vi "movimentacao_cin_inv_bezier_2.vi"() -> ()   [LabVIEW 2017]
doc: "The myRIO Project template acquires acceleration data from the onboard accelerometer and displays the changes of acceleration values in a waveform chart."
uses:
  <vilib>/Analysis/Matrix/Datatypes/RealMatrix.ctl
  <vilib>/myRIO/Instrument Drivers/Onboard IO/I2C/typedefs/I2C User Configuration.ctl
  <vilib>/myRIO/Instrument Drivers/Onboard IO/I2C/typedefs/I2C Transfer Rate.ctl
  <vilib>/myRIO/Instrument Drivers/Onboard IO/PWM/typedefs/PWM Reference.ctl
  <vilib>/myRIO/Common/Instrument Driver Framework/Utilities/typedefs/myRIO Generic Hardware Reference.ctl
  <vilib>/myRIO/Common/Instrument Driver Framework/Utilities/typedefs/Hardware Version Enum.ctl
  <vilib>/myRIO/Common/Instrument Driver Framework/Utilities/typedefs/myRIO v1.0 Reference.ctl
  <vilib>/myRIO/Common/Instrument Driver Framework/Utilities/typedefs/Generic FPGA Reference.ctl
  <vilib>/myRIO/Common/Instrument Driver Framework/myRIO v1.0/PWM/typedefs/PWM Channels Enum.ctl
  <vilib>/myRIO/Instrument Drivers/Onboard IO/PWM/typedefs/PWM Configuration.ctl
  <vilib>/userdefined/High Color/nirio_resource_hc.ctl
  <vilib>/myRIO/Instrument Drivers/Onboard IO/I2C/typedefs/I2C Reference.ctl
  <vilib>/myRIO/Common/Instrument Driver Framework/myRIO v1.0/I2C/typedefs/I2C Channels Enum.ctl
  <vilib>/myRIO/Instrument Drivers/Onboard IO/I2C/typedefs/I2C Configuration.ctl
  <vilib>/myRIO/Common/Instrument Driver Framework/myRIO v1.0/I2C/vis/myRIO v1.1 Open I2C.vi
  <vilib>/myRIO/Common/Instrument Driver Framework/myRIO v1.0/PWM/vis/myRIO v1.1 Open PWM.vi
  <vilib>/myRIO/Common/Instrument Driver Framework/Utilities/vis/Validate Channels.vi
  <vilib>/myRIO/Common/Instrument Driver Framework/myRIO v1.0/I2C/vis/myRIO v1.0 Reserve I2C.vi
  <vilib>/myRIO/Common/Instrument Driver Framework/myRIO v1.0/PWM/vis/myRIO v1.0 Reserve PWM.vi
  <vilib>/myRIO/Instrument Drivers/Onboard IO/PWM/vis/Set Duty Cycle and Frequency.vi
  <vilib>/myRIO/Common/Instrument Driver Framework/myRIO v1.0/I2C/vis/myRIO v1.0 Close I2C.vi
  <vilib>/myRIO/Common/Instrument Driver Framework/myRIO v1.0/PWM/vis/myRIO v1.0 Close PWM.vi
  <vilib>/myRIO/Common/Instrument Driver Framework/myRIO v1.0/I2C/vis/myRIO v1.0 Build MUX Configuration I2C.vi
  <vilib>/myRIO/Common/Instrument Driver Framework/myRIO v1.0/Resource Manager/vis/myRIO v1.0 Reserve Channel List.vi
  <vilib>/myRIO/Common/Instrument Driver Framework/myRIO v1.0/PWM/vis/myRIO v1.0 Build MUX Configuration PWM.vi
  <vilib>/myRIO/Common/Instrument Driver Framework/myRIO v1.0/I2C/vis/myRIO v1.0 Unreserve I2C.vi
  <vilib>/myRIO/Common/Instrument Driver Framework/myRIO v1.0/PWM/vis/myRIO v1.0 Unreserve PWM.vi
  <vilib>/myRIO/Common/Instrument Driver Framework/myRIO v1.0/Resource Manager/vis/myRIO v1.0 Create Configuration List.vi
  <vilib>/myRIO/Common/Instrument Driver Framework/myRIO v1.0/Resource Manager/vis/myRIO v1.0 Reserve Channel.vi
  <vilib>/myRIO/Common/Instrument Driver Framework/myRIO v1.0/Resource Manager/vis/myRIO v1.0 Unreserve Channel.vi
  <vilib>/myRIO/Common/Instrument Driver Framework/myRIO v1.0/Resource Manager/vis/myRIO v1.0 Unreserve Channel List.vi
  <vilib>/myRIO/Common/Instrument Driver Framework/myRIO v1.0/Resource Manager/vis/myRIO v1.0 Build Mutex Name.vi
  <vilib>/Utility/VariantDataType/GetNumericInfo.vi
  <vilib>/Utility/error.llb/Error Cluster From Error Code.vi
  <vilib>/myRIO/Common/Instrument Driver Framework/myRIO v1.0/myRIO v1.1 Open.vi
  <vilib>/myRIO/Common/Instrument Driver Framework/Utilities/vis/IO Manager.vi
  <vilib>/myRIO/Common/Instrument Driver Framework/Utilities/vis/Configuration Manager.vi
  <vilib>/myRIO/Common/Instrument Driver Framework/myRIO v1.0/Resource Manager/vis/myRIO v1.0 Configure IO.vi
  <vilib>/myRIO/Common/Instrument Driver Framework/myRIO v1.0/myRIO v1.0 Close.vi
  <vilib>/myRIO/Common/Instrument Driver Framework/myRIO v1.0/PWM/vis/myRIO v1.0 Write PWM.vi
  <vilib>/myRIO/Common/Instrument Driver Framework/myRIO v1.0/I2C/vis/myRIO v1.0 Configure I2C.vi
  <vilib>/myRIO/Common/Instrument Driver Framework/myRIO v1.0/I2C/vis/myRIO v1.0 Shutdown I2C.vi
  <vilib>/myRIO/Common/Instrument Driver Framework/myRIO v1.0/PWM/vis/myRIO v1.0 Shutdown PWM.vi
  <vilib>/myRIO/Instrument Drivers/Onboard IO/PWM/vis/myRIO PWM Open.xnode
  <vilib>/myRIO/Instrument Drivers/Onboard IO/I2C/vis/myRIO I2C Open.xnode
  <vilib>/myRIO/Instrument Drivers/Onboard IO/PWM/PWM.lvlib
  <vilib>/myRIO/Instrument Drivers/Onboard IO/I2C/I2C.lvlib
  <vilib>/Analysis/Matrix/NI_Matrix.lvlib
panel:
  out "Range":u16
  out "Waveform Chart":u16(graph)
  out "Objeto":bool
  out "did_timeout":bool
  out "dt":u32
  out "distancaia":dbl format="%0.2f"
  out "error out":errorcluster
  out "init status":bool
  out "Objeto detectado 2":bool
  out "Parar_esteira":bool
  out "result string":string
  out "iterador":u32
  out "number of rows":i32
  out "matrix":T1
  in  "Ring":u16(ring) items=["A", "B", "C"]
  out "x .and. y?":bool
  in  "OK Button":bool
  out "subarray":dbl[](array[numeric])
  out "appended array 2":dbl[](array[numeric])
  out "logical AND":bool
  out "x = y?":bool[](array[boolean])
  out "POS_E_ORIEN_HOME":dbl[](array[numeric])
  out "ANG_POSI_E_ORIEN_HOME":dbl[](array[numeric])
  out "CURRENT POSITIONS OF THE MOTORS":dbl[](array[numeric])
  in  "angulo_garra":dbl(knob) scale=-180.0..180.0
  in  "Duty Cycle Abert":dbl=0.04 format="%#_13g"
  out "Actuator 2":bool
  in  "Actuator":bool
  in  "Conveyor speed (mm/s)":dbl(slide)=200.0 step=1.0 scale=0.0..350.0
  out "indexador":i32
  out "Objeto detectado":bool
  out "Manipulando":bool
  out "Está em Home":bool
  out "Posicao_desejada":bool
  in  "Home":bool
  in  "error in (no error)":errorcluster
  in  "PARAR":bool
  in  "POSITION VECTOR":dbl[](array[numeric])
  # "ROTINA DE CONTROLE DO PROTÓTIPO DE FMS"
  # "COMANDO DE POSIÇÃO\nATUAL DOS MOTORES"
  # "OPERATION STATUS"
  # "ÂNGULOS DE JUNTAS"
  # "THETA 1"
  # "MOTOR 1"
  # "HOME"
  # "THETA 2"
  # "MOTOR 2"
  # "DESIRED POSITION"
  # "THETA 3"
  # "MOTOR 3"
  # "OBJECT DETECTED"
  # "THETA 4"
  # "MOTOR 4"
  # "MANIPULATING"
  # "THETA 5"
  # "MOTOR 5"
  # "ACTUATOR"
  # "MOTOR 6"
  # "VELOCIDADE DA ESTEIRA (mm/s)"
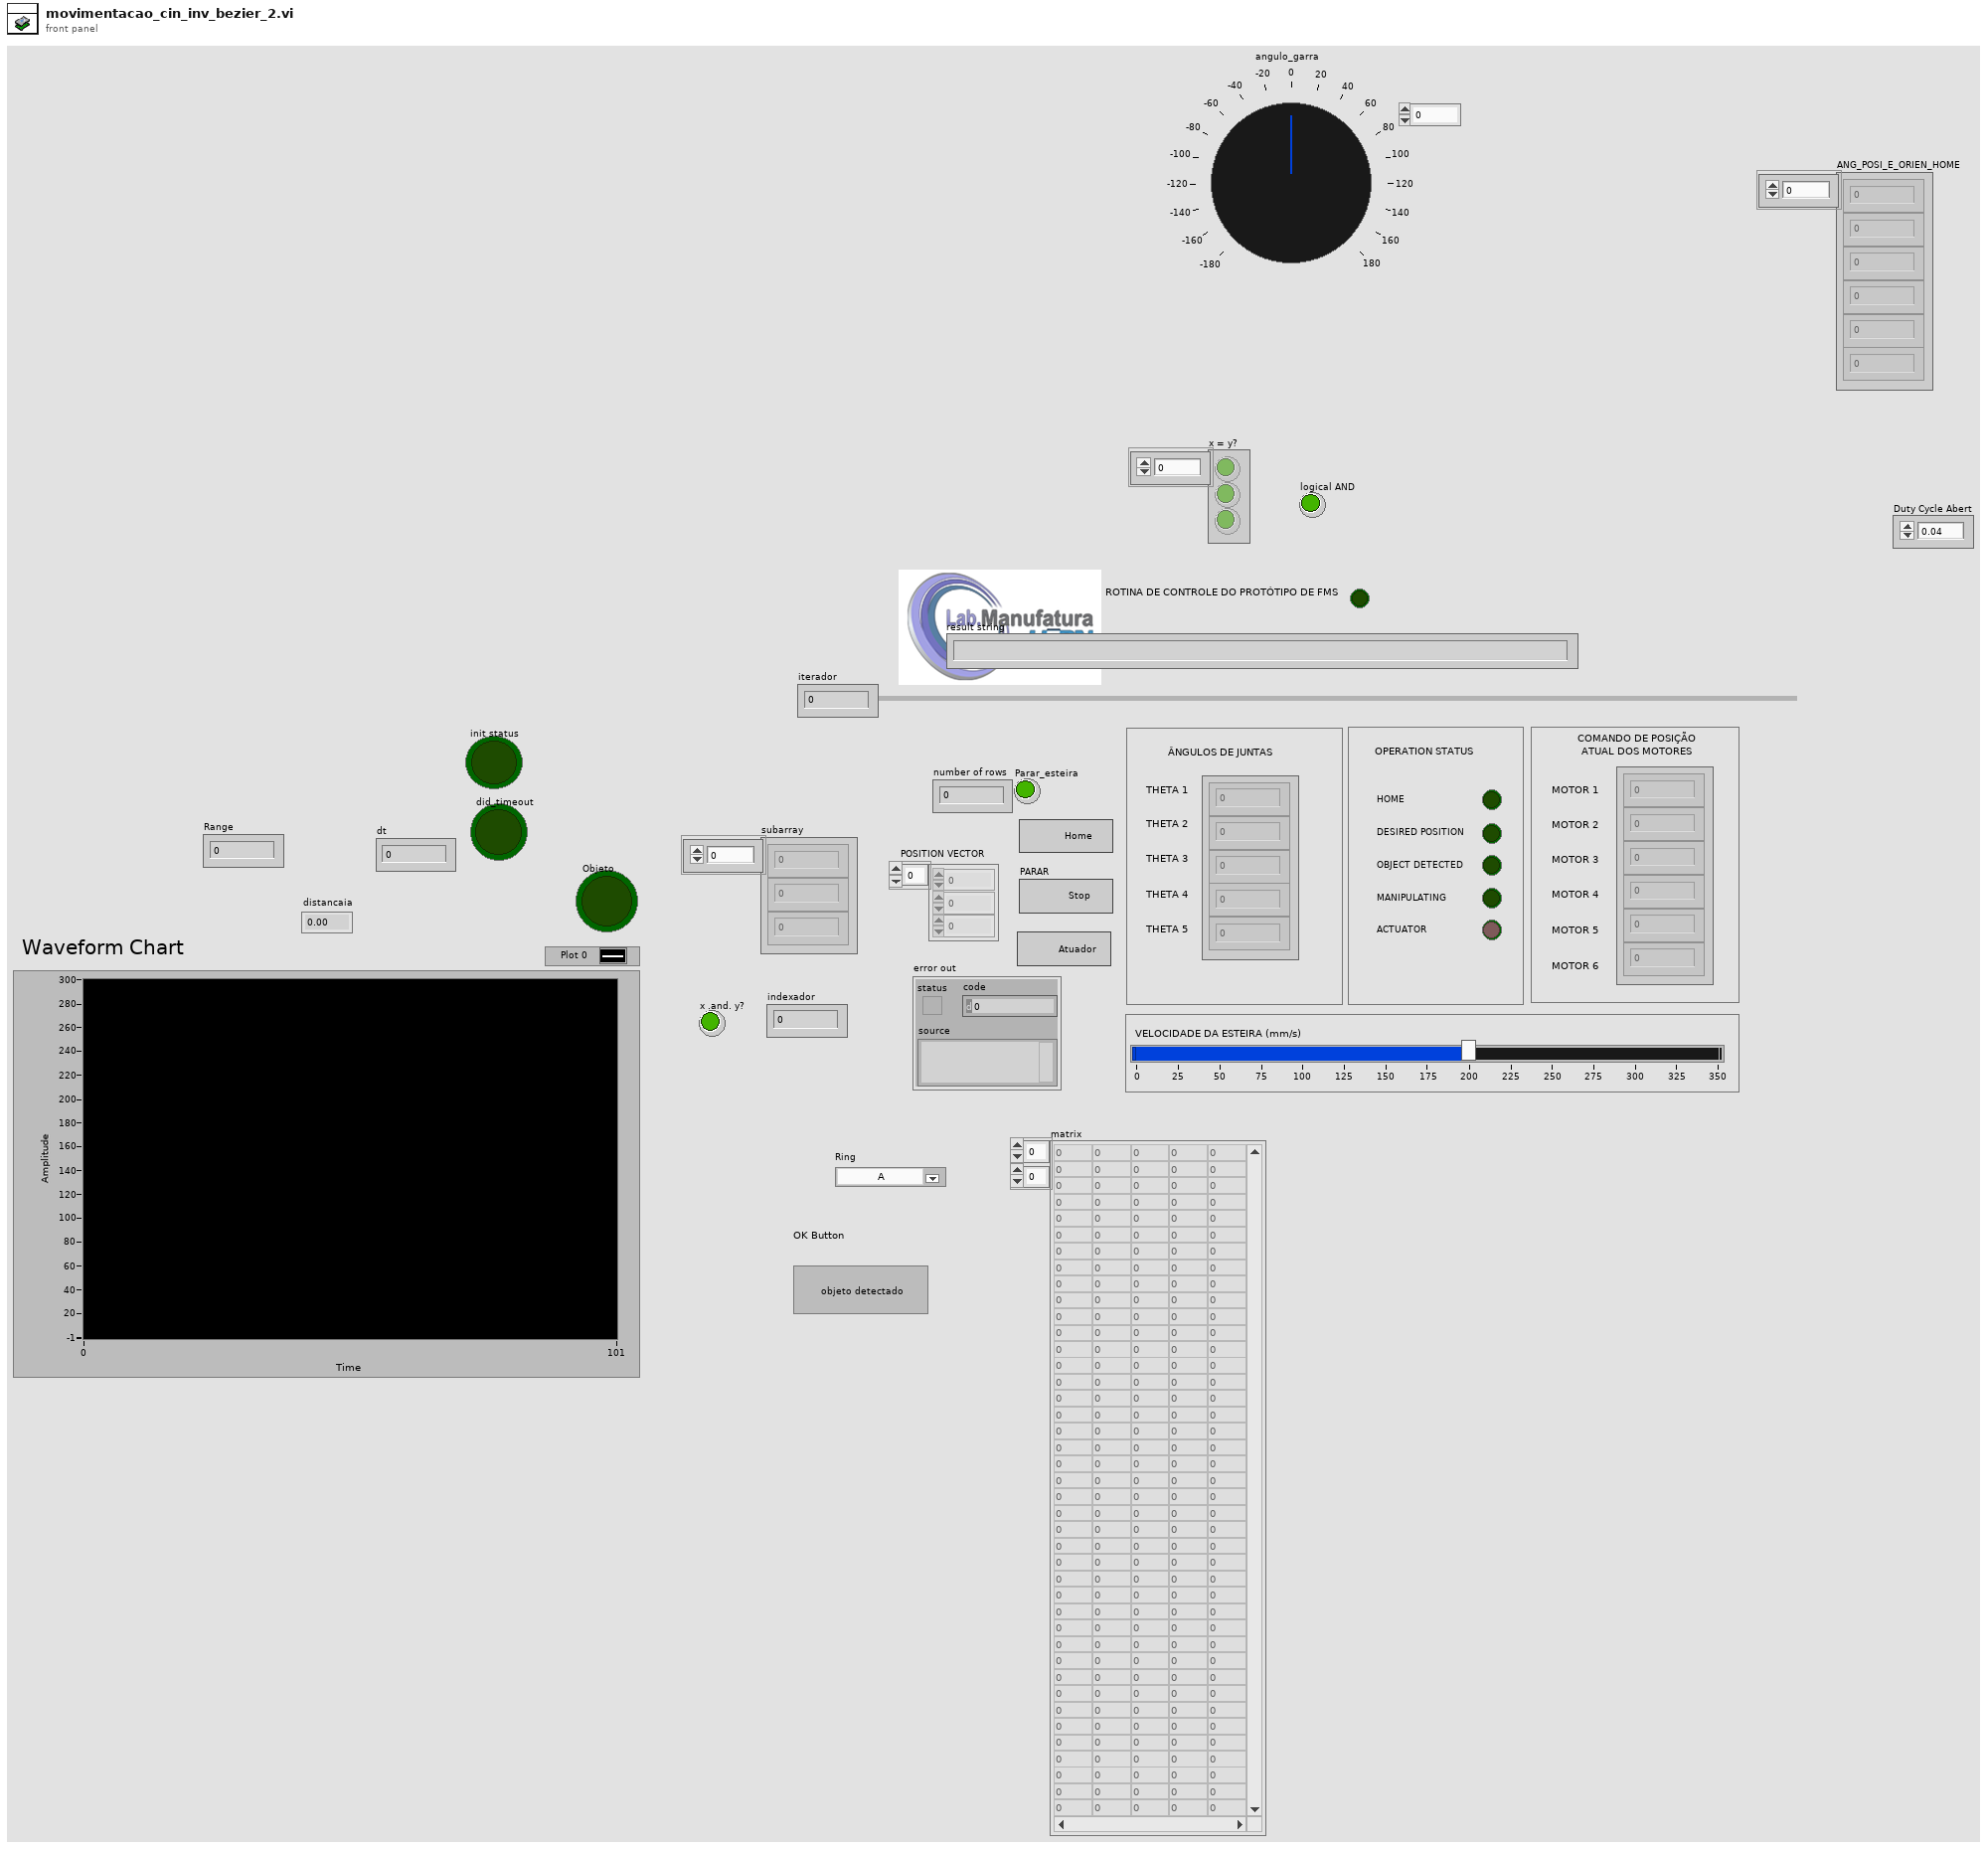
[diagram p1: front panel]
types:
  T1 = typedef "NI_Matrix.lvlib/RealMatrix.ctl" = dbl[][]
  T2 = typedef "I2C.lvlib/I2C User Configuration.ctl" = cluster{"I2C Transfer Rate":T3}
  T3 = typedef "I2C.lvlib/I2C Transfer Rate.ctl" = enum16{"Standard mode (100 kbps)", "Fast mode (400 kbps)"}
  T4 = cluster{"theta 1":dbl, "theta 2":dbl, "theta 3":dbl, "theta5":dbl, "theta4":dbl}
  T5 = typedef "I2C.lvlib/I2C Reference.ctl" = cluster{"myRIO Reference":T6, "I2C Channels Enum":T10, "I2C Configuration":T11}
  T6 = typedef "myRIO Generic Hardware Reference.ctl" = cluster{"myRIO Model":T7, "myRIO Hardware Reference":T8}
  T7 = typedef "Hardware Version Enum.ctl" = enum16{"Unknown", "myRIO-1900", "myRIO-1950", "roboRIO", "NI ELVIS RIO CM"}
  T8 = typedef "myRIO v1.0 Reference.ctl" = cluster{"Generic FPGA Reference":T9, "Allow multiple opens":bool}
  T9 = typedef "Generic FPGA Reference.ctl" = refnum<k20>
  T10 = typedef "I2C Channels Enum.ctl" = enum16{"Not Connected", "A/I2C", "B/I2C", "I2C/I2C"}
  T11 = typedef "I2C.lvlib/I2C Configuration.ctl" = cluster{"I2C Transfer Rate":T3}
  T12 = typedef "nirio_resource_hc.ctl" = tag
  T13 = typedef "PWM.lvlib/PWM Reference.ctl" = cluster{"myRIO Reference":T6, "PWM Channels Enum":T14, "PWM Configuration":T15}
  T14 = typedef "PWM Channels Enum.ctl" = enum16{"Not Connected", "C/PWM0", "C/PWM1", "A/PWM0", "A/PWM1", "A/PWM2", "B/PWM0", "B/PWM1", "B/PWM2", "PWM/PWM0", "PWM/PWM1", "PWM/PWM2", "PWM/PWM3", "PWM/PWM4", "PWM/PWM5", "PWM/PWM6", "PWM/PWM7", "PWM/PWM8", "PWM/PWM9"}
  T15 = typedef "PWM.lvlib/PWM Configuration.ctl" = cluster{"Frequency":dbl, "Duty Cycle":dbl}
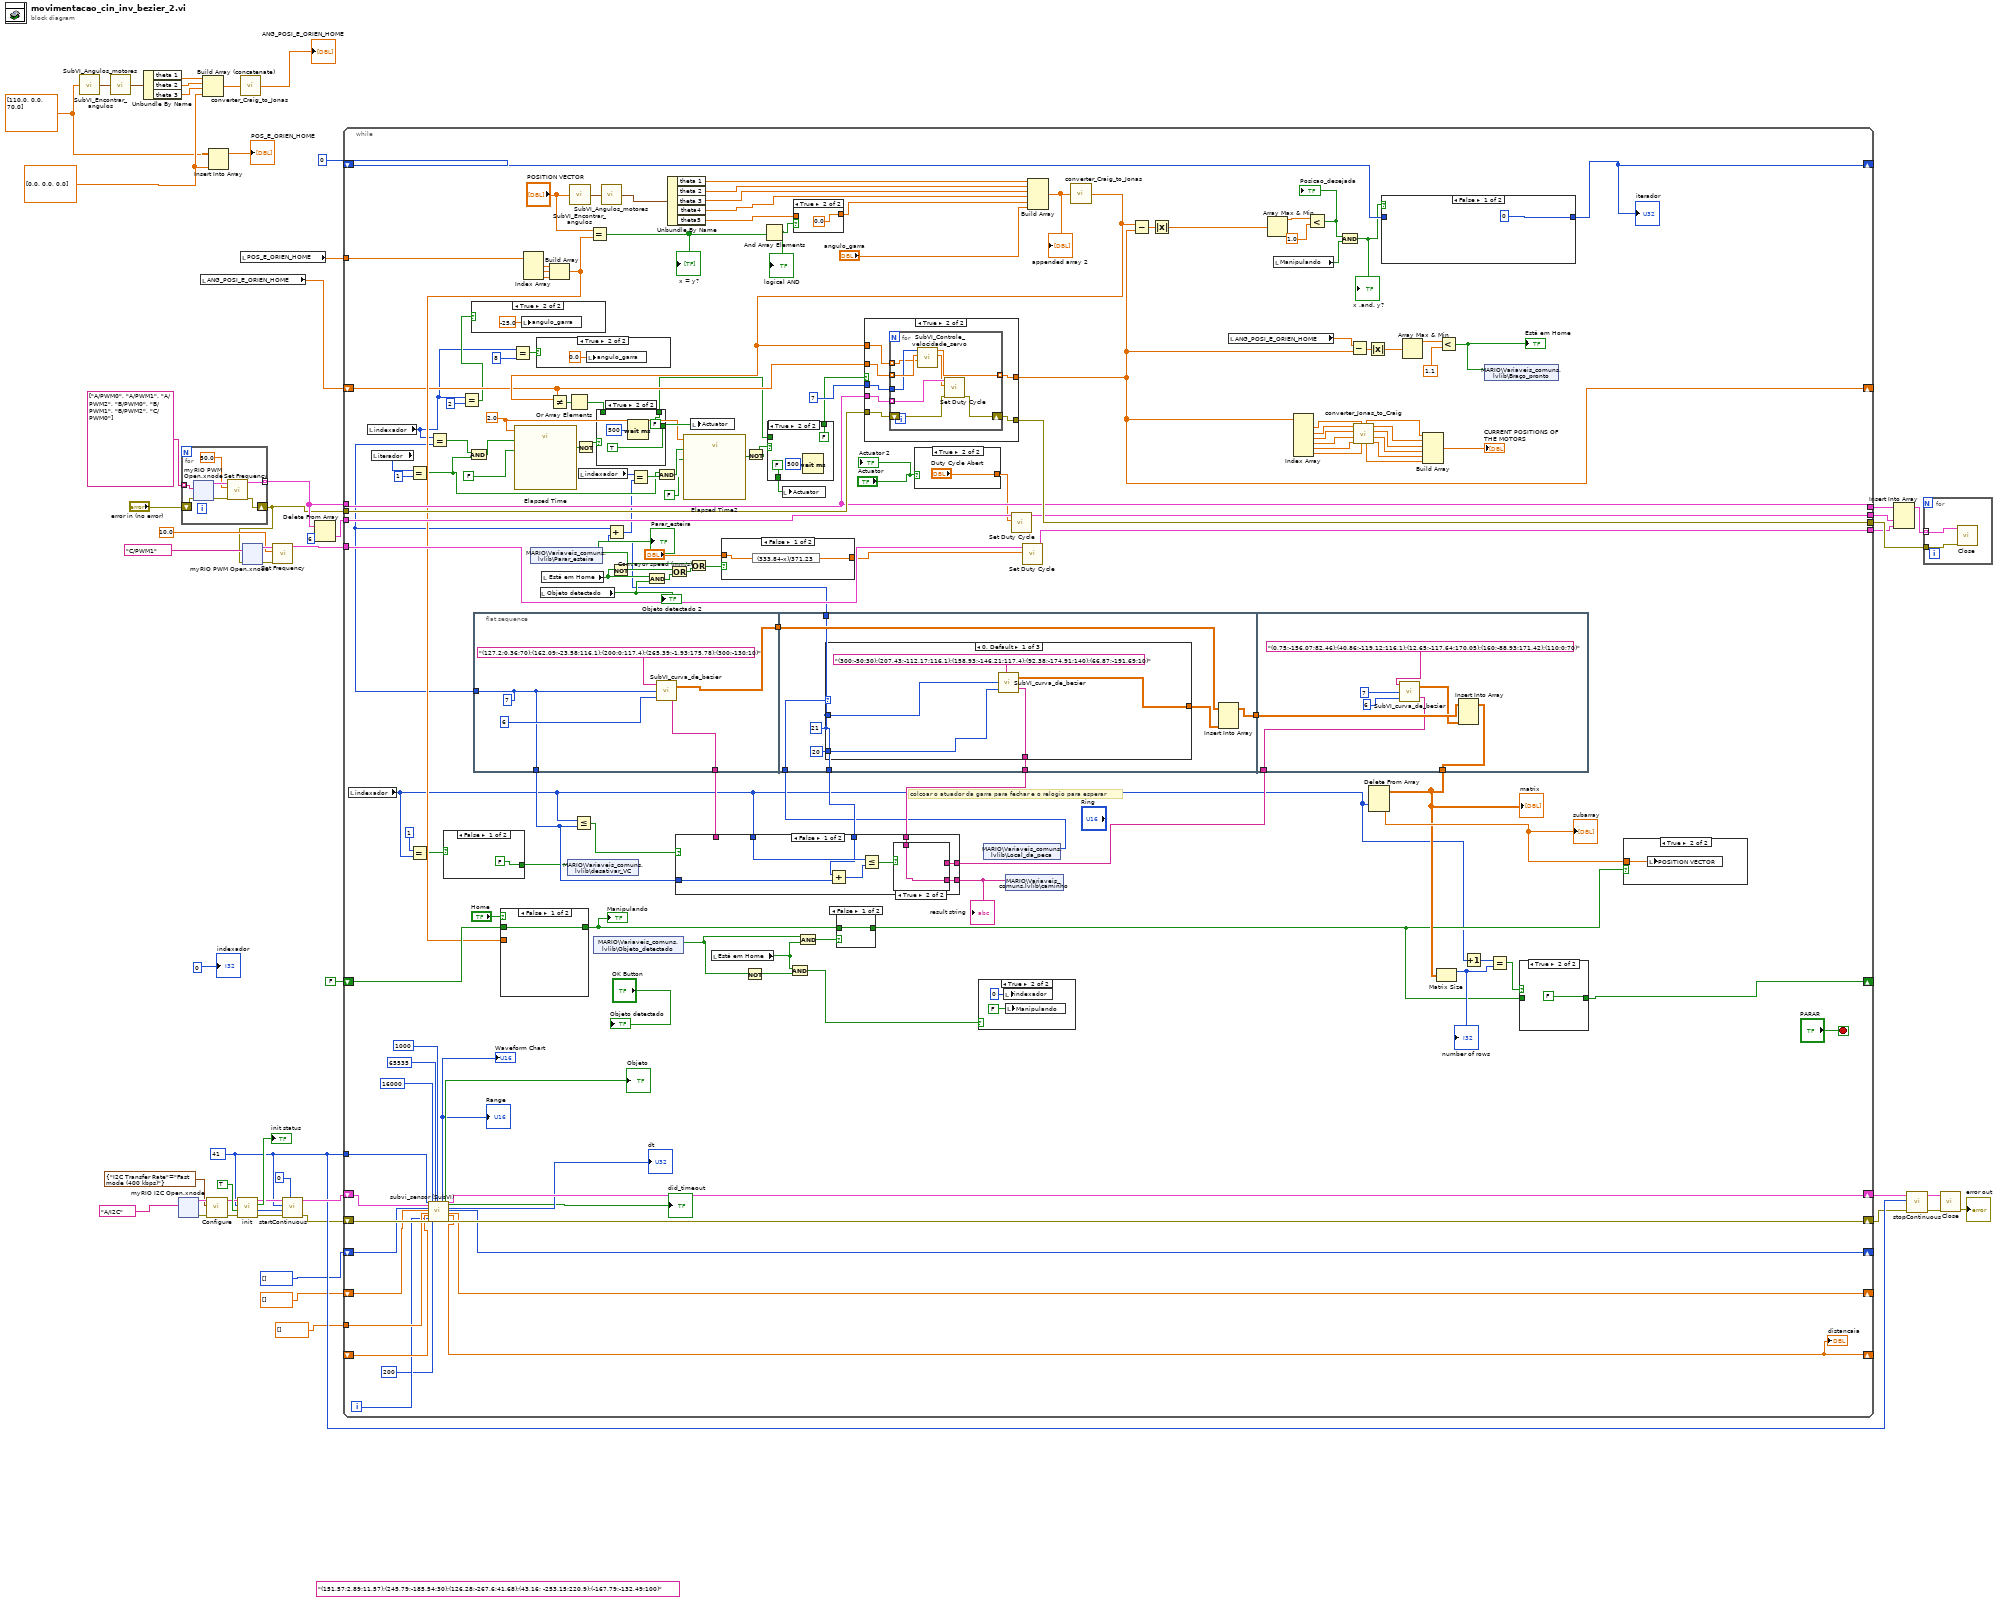
[diagram p0: block diagram]
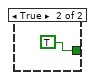
[diagram p2: hidden frame]
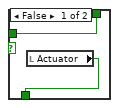
[diagram p7: hidden frame]
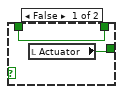
[diagram p8: hidden frame]
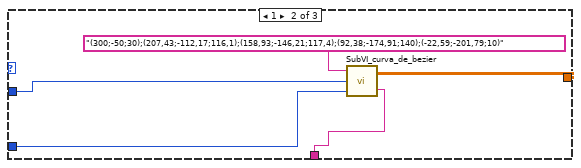
[diagram p10: hidden frame]
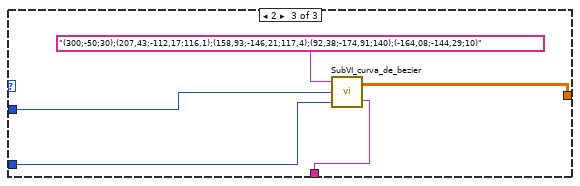
[diagram p11: hidden frame]
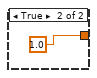
[diagram p12: hidden frame]
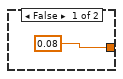
[diagram p13: hidden frame]
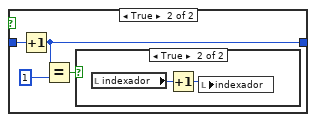
[diagram p16: hidden frame]
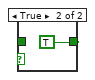
[diagram p19: hidden frame]
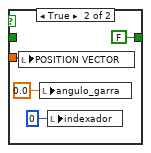
[diagram p20: hidden frame]
diagram:
  w9 = u8 41
  (unwired) "(151,57;2,89;11,57);(245,79;-185,54;30);(126,28;-267,6;41,68);(43,16; -253,15;220,9);(-167,79;-132,49;100)" ("String 2")
  w31 = dbl[] [0.0, 0.0, 0.0] ("vetor_P")
  w26 = dbl[] [110.0, 0.0, 70.0] ("vetor_P")
  n1 = call "SubVI_Encontrar_angulos.vi"("vetor_P"=w26) -> ("ângulos de Juntas"=w25:T4)
  n2 = call "SubVI_Angulos_motores.vi"("input cluster"=w25) -> ("output cluster"=w24:T4)
  n3 = Unbundle By Name(w24) -> ("theta 1"=w35:dbl, "theta 2"=w34:dbl, "theta 3"=w33:dbl)
  n4 = xnode "myRIO I2C Open.xnode"("Channel Name"=tag "A/I2C") -> ("error out"=w22:errorcluster, "I2C Ref Out"=w23:T5)  [unwired: 2 in]
  n5 = for {
    tunnel: tag[] ["A/PWM0", "A/PWM1", "A/PWM2", "B/PWM0", "B/PWM1", "B/PWM2", "C/PWM0"] -> [w58] mode=indexing
    tunnel: [w57] -> w48 mode=indexing
    shift-right: [w56] -> w37
    shift-left: "error in (no error)" -> [w55]
    n6 = xnode ("myRIO PWM Open.xnode")("error in (no error)"=w55, "Channel Name"=w58) -> ("error out"=w59:errorcluster, "PWM Ref Out"=w61:T13)  [unwired: 1 in]
    n7 = call <vilib>:"Set Frequency.vi"("error in (no error)"=w59, "Frequency [Hz]"=50.0, "PWM Ref In"=w61) -> ("error out"=w56:errorcluster, "PWM Ref Out"=w57:T13)  [unwired: 6 in]
  }
  n8 = local read "ANG_POSI_E_ORIEN_HOME"() -> (w32:dbl[])
  n9 = Build Array (concatenate)(w35, w34, w33, w31) -> (w28:dbl[])
  n10 = call <vilib>:"Configure.vi"("error in (no error)"=w22, "I2C User Configuration"=T2 {"I2C Transfer Rate"=enum."Fast mode (400 kbps)"}, "I2C Ref In"=w23) -> ("error out"=w17:errorcluster, "I2C Ref Out"=w18:T5)  [unwired: 7 in]
  n11 = Insert Into Array(array=w26, new element=w31) -> (→"POS_E_ORIEN_HOME":dbl[])  [unwired: 1 in]
  n12 = call "init.vi"("error in"=w17, "io_2V8"=TRUE, "Slave Address(7 bit)"=w9, "I2C Ref In"=w18) -> ("error out"=w14:errorcluster, "stop_variable"=w13:u8, "Boolean"=→"init status":bool, "I2C Ref Out"=w15:T5)  [unwired: 4 in]
  n13 = call "converter_Craig_to_Jonas.vi"("array"=w28) -> ("appended array"=→"ANG_POSI_E_ORIEN_HOME":dbl[])
  n14 = local read "POS_E_ORIEN_HOME"() -> (w29:dbl[])
  n15 = xnode "myRIO PWM Open.xnode"("error in (no error)"=w37, "Channel Name"=tag "C/PWM1") -> ("error out"=w41:errorcluster, "PWM Ref Out"=w42:T13)  [unwired: 1 in]
  n16 = call <vilib>:"Set Frequency.vi"("error in (no error)"=w41, "Frequency [Hz]"=10.0, "PWM Ref In"=w42) -> ("PWM Ref Out"=w38:T13)  [unwired: 6 in, 1 out]
  n17 = call "startContinuous.vi"("period_ms"=u32 0, "error in"=w14, "stop_variable"=w13, "Slave Address(7 bit)"=w9, "I2C Ref In"=w15) -> ("error out"=w4:errorcluster, "I2C Ref Out"=w11:T5)  [unwired: 5 in]
  n18 = Delete From Array(array=w48, index=6) -> (deleted portion=w46:T13)  [unwired: 1 in, 1 out]
  n19 = while {
    tunnel: [w225] -> w54
    shift-right: [w157] -> _
    shift-left: w32 -> [w149]
    tunnel: w37 -> [w223]
    tunnel: w48 -> [w222]
    tunnel: [w222] -> w45
    shift-right: [w143] -> _
    shift-left: FALSE -> [w206]
    shift-right: [w215] -> _
    shift-left: u32 0 ("ms to wait (braço)") -> [w214]
    tunnel: w46 -> [w201]
    tunnel: [w200] -> w44
    tunnel: w38 -> [w198]
    tunnel: [w194] -> w36
    tunnel: w29 -> [w164]
    tunnel: w9 -> [w98]
    shift-right: [w97] -> w10
    shift-left: w11 -> [w96]
    shift-right: [w95] -> w5
    shift-left: w4 -> [w94]
    shift-right: [w93] -> _
    shift-left: u16[] [] -> [w92]
    shift-right: [w91] -> _
    shift-left: dbl[] [] ("array") -> [w90]
    tunnel: dbl[] [] ("array") -> [w89]
    shift-right: [w87] -> _
    shift-left: _ -> [w88]
    i -> [w86]
    stop <- "PARAR" stop-if-true
    w127 = 2.0 ("Time Target (s)")
    # "colcoar o atuador da garra para fechar e o relogio para esperar"
    n20 = local read "indexador"() -> (w104:i32)
    n21 = local read "indexador"() -> (w106:i32)
    n22 = local read "iterador"() -> (w140:u32)
    n23 = Equal?(x=w140, y=u32 1) -> (x = y?=w129:bool)
    n24 = Equal?(x=1, y=w104) -> (x = y?=w102:bool)
    n25 = call "subvi_sensor (SubVI).vi"("Numeric Control 2"=w98, "I2C Ref Out in"=w96, "Array in"=w92, "array in"=w90, "array 3"=w89, "mean in"=w88, "Numeric Control 3"=w86, "error in (no error)"=w94, "io_timeout"=u16 16000, "Numeric Control"=200, "y 2"=u16 65535 ("y"), "y"=u16 1000) -> ("Range"=→"Waveform Chart" →"Range":u16, "Boolean"=→"Objeto":bool, "I2C Ref Out out"=w97:T5, "did_timeout"=→"did_timeout":bool, "Numeric Control 4"=→"dt":u32, "Array out"=w93:u16[], "array out"=w91:dbl[], "mean out"=w87:dbl, "error out"=w95:errorcluster)  [unwired: 7 in]
    "distancaia" <- w87
    n26 = Equal?(x=w106, y=w118) -> (x = y?=w132:bool)
    n27 = case shown="False" w102 {
      tunnel: [FALSE TRUE] -> w101
      frame False {
      }
      frame True {
      }
    }
    n28 = Equal?(x=w106, y=2) -> (x = y?=w109:bool)
    n29 = And(x=w132, y=w129) -> (x .and. y?=w138:bool)
    n30 = case shown="True" w109 {
      frame False {
      }
      frame True {
        n31 = local write "angulo_garra"(-25.0 ("angulo_garra")) -> ()
      }
    }
    n32 = flat-sequence {
      tunnel: [w256] -> w146
      tunnel: [w254] -> w118
      tunnel: [w254] -> w111
      tunnel: [w253] -> w116
      tunnel: w146 -> [w263]
      tunnel: [w264] -> w145
      tunnel: [w259] -> w119
      tunnel: w105 -> [w260]
      tunnel: [w259] -> w115
      tunnel: [w258] -> w113
      tunnel: [w281] -> w144
      tunnel: w145 -> [w283]
      tunnel: [w280] -> w112
      frame #0 {
        w254 = i64 7 ("número de pontos que a matriz deve retornar (nº de divisões + 1)")
        n33 = call "SubVI_curva_de_bezier.vi"("Nº de divisões da curva de Bézier (padrão: 20 divisões = 21 pontos)"=6, "número de pontos que a matriz deve retornar (padrão: nº de divisões + 1)"=w254, "String in"="(127,2;0,36;70);(162,09;-23,58;116,1);(200;0;117,4);(265,39;-1,93;175,78);(300;-130;10)" ("Esteira")) -> ("result string"=w253:string, "matrix"=w256:T1)
      }
      frame #1 {
        w259 = i64 21 ("número de pontos que a matriz deve retornar (nº de divisões + 1)")
        n34 = case shown="0, Default" w260 {
          tunnel: [w269 w274 w279] -> w262
          tunnel: w259 -> [w267 w273 w277]
          tunnel: 20 ("Nº de divisões da curva de Bézier (padrão: 20 divisões = 21 pontos)") -> [w266 w272 w276]
          tunnel: [w265 w270 w275] -> w258
          frame 0, Default {
            n35 = call "SubVI_curva_de_bezier.vi"("Nº de divisões da curva de Bézier (padrão: 20 divisões = 21 pontos)"=w266, "número de pontos que a matriz deve retornar (padrão: nº de divisões + 1)"=w267, "String in"="(300;-50;30);(207,43;-112,17;116,1);(158,93;-146,21;117,4);(92,38;-174,91;140);(66,87;-191,69;10)" ("Esteira")) -> ("result string"=w265:string, "matrix"=w269:T1)
          }
          frame 1 {
            n36 = call "SubVI_curva_de_bezier.vi"("Nº de divisões da curva de Bézier (padrão: 20 divisões = 21 pontos)"=w272, "número de pontos que a matriz deve retornar (padrão: nº de divisões + 1)"=w273, "String in"="(300;-50;30);(207,43;-112,17;116,1);(158,93;-146,21;117,4);(92,38;-174,91;140);(-22,59;-201,79;10)" ("Esteira")) -> ("result string"=w270:string, "matrix"=w274:T1)
          }
          frame 2 {
            n37 = call "SubVI_curva_de_bezier.vi"("Nº de divisões da curva de Bézier (padrão: 20 divisões = 21 pontos)"=w276, "número de pontos que a matriz deve retornar (padrão: nº de divisões + 1)"=w277, "String in"="(300;-50;30);(207,43;-112,17;116,1);(158,93;-146,21;117,4);(92,38;-174,91;140);(-164,08;-144,29;10)" ("Esteira")) -> ("result string"=w275:string, "matrix"=w279:T1)
          }
        }
        n38 = Insert Into Array(array=w263, new element=w262) -> (w264:T1)  [unwired: 2 in]
      }
      frame #2 {
        n39 = call "SubVI_curva_de_bezier.vi"("Nº de divisões da curva de Bézier (padrão: 20 divisões = 21 pontos)"=6, "número de pontos que a matriz deve retornar (padrão: nº de divisões + 1)"=i64 7 ("número de pontos que a matriz deve retornar (nº de divisões + 1)"), "String in"="(0,75;-156,07;82,46);(40,86;-119,12;116,1);(12,65;-117,64;170,05);(160;-88,93;171,42);(110;0;70)" ("Esteira")) -> ("result string"=w280:string, "matrix"=w282:T1)
        n40 = Insert Into Array(array=w283, new element=w282) -> (w281:T1)  [unwired: 2 in]
      }
    }
    n41 = Equal?(x=w106, y=8) -> (x = y?=w107:bool)
    n42 = call "Elapsed Time"("Time Target (s)"=w127, "Reset"=w138, "Auto Reset"=FALSE) -> ("Time has Elapsed"=w136:bool)  [unwired: 9 in, 7 out]
    n43 = Index Array(array=w164) -> (element #1=w167:dbl, element #2=w166:dbl, element #3=w165:dbl)  [unwired: 3 in]
    n44 = shared-variable "MARIO\\Variaveis_comuns.lvlib\\Parar_esteira"() -> (w193:bool)  [unwired: 1 in, 1 out]
    "Parar_esteira" <- w193
    n45 = case shown="True" w107 {
      frame False {
      }
      frame True {
        n46 = local write "angulo_garra"(0.0 ("angulo_garra")) -> ()
      }
    }
    n47 = local read "Objeto detectado"() -> (w191:bool)
    "Objeto detectado 2" <- w191
    n48 = local read "Está em Home"() -> (w188:bool)
    n49 = Build Array(w167, w166, w165) -> (w163:dbl[])
    n50 = case shown="False" "Home" {
      tunnel: w163 -> [_ w311]
      tunnel: w206 -> [w307 _]
      tunnel: [w307 FALSE ("Manipulando")] -> w156
      frame False {
      }
      frame True {
        n51 = local write "POSITION VECTOR"(w311) -> ()
        n52 = local write "angulo_garra"(0.0 ("angulo_garra")) -> ()
        n53 = local write "indexador"(0 ("indexador")) -> ()
      }
    }
    "Manipulando" <- w156
    n54 = shared-variable "MARIO\\Variaveis_comuns.lvlib\\desativar_VC"(w101) -> ()  [unwired: 1 in, 1 out]
    n55 = call "SubVI_Encontrar_angulos.vi"("vetor_P"="POSITION VECTOR") -> ("ângulos de Juntas"=w154:T4)
    n56 = Less Or Equal?(x=w104, y=w111) -> (x <= y?=w117:bool)
    n57 = Not(x=w136) -> (.not. x?=w135:bool)
    n58 = local read "indexador"() -> (w131:i32)
    n59 = Equal?(x="POSITION VECTOR", y=w163) -> (x = y?=w204:bool[])
    "x = y?" <- w204
    n60 = shared-variable "MARIO\\Variaveis_comuns.lvlib\\Objeto_detectado"() -> (w99:bool)  [unwired: 1 in, 1 out]
    n61 = call "SubVI_Angulos_motores.vi"("input cluster"=w154) -> ("output cluster"=w153:T4)
    n62 = Add(x=w118, y=w119) -> (x+y=w120:i64)
    n63 = Not(x=w188) -> (.not. x?=w189:bool)
    n64 = Equal?(x=w131, y=w120) -> (x = y?=w130:bool)
    n65 = And(x=w188, y=w191) -> (x .and. y?=w190:bool)
    n66 = And(x=w129, y=w130) -> (x .and. y?=w128:bool)
    n67 = Unbundle By Name(w153) -> ("theta 1"=w173:dbl, "theta 2"=w172:dbl, "theta 3"=w171:dbl, "theta4"=w152:dbl, "theta5"=w151:dbl)
    n68 = Or(x=w189, y=w190) -> (x .or. y?=w187:bool)
    n69 = case shown="False" w117 {
      tunnel: w116 -> [_ w241]
      tunnel: w104 -> [w238 _]
      tunnel: w115 -> [w233 _]
      tunnel: [w236 w241] -> w114
      tunnel: w113 -> [w235 _]
      tunnel: w112 -> [w234 _]
      tunnel: w111 -> [w232 _]
      frame False {
        n70 = Add(x=w233, y=w232) -> (x+y=w231:i64)
        n71 = Less Or Equal?(x=w238, y=w231) -> (x <= y?=w237:bool)
        n72 = case shown="True" w237 {
          tunnel: [w239 w240] -> w236
          tunnel: w235 -> [_ w240]
          tunnel: w234 -> [w239 _]
          frame False {
          }
          frame True {
          }
        }
      }
      frame True {
      }
    }
    "result string" <- w114
    n73 = call "Elapsed Time2"("Time Target (s)"=w127, "Reset"=w128, "Auto Reset"=FALSE) -> ("Time has Elapsed"=w126:bool)  [unwired: 9 in, 7 out]
    n74 = Or(x=w193, y=w187) -> (x .or. y?=w195:bool)
    n75 = local read "Está em Home"() -> (w160:bool)
    n76 = case shown="False" w195 {
      tunnel: [w288 1.0 ("Duty Cycle")] -> w197
      tunnel: "Conveyor speed (mm/s)" -> [w287 _]
      frame False {
        n77 = expression code="(333.84-x)/371.23"(w287) -> (w288:dbl)
      }
      frame True {
      }
    }
    n78 = Not(x=w99) -> (.not. x?=w159:bool)
    n79 = Not(x=w126) -> (.not. x?=w125:bool)
    n80 = And Array Elements(Boolean array=w204) -> (logical AND=w203:bool)
    "logical AND" <- w203
    n81 = And(x=w160, y=w159) -> (x .and. y?=w211:bool)
    n82 = case shown="True" w203 {
      tunnel: [w292 0.0 ("theta5")] -> w170
      tunnel: w151 -> [w292 _]
      frame False {
      }
      frame True {
      }
    }
    n83 = And(x=w99, y=w160) -> (x .and. y?=w217:bool)
    n84 = case shown="False" w217 {
      tunnel: [w305 TRUE] -> w141
      tunnel: w156 -> [w305 _]
      frame False {
      }
      frame True {
      }
    }
    n85 = case shown="True" "Actuator" {
      tunnel: [0.08 ("Duty Cycle Abert") "Duty Cycle Abert"] -> w199
      frame False {
      }
      frame True {
      }
    }
    n86 = case shown="True" w211 {
      frame False {
      }
      frame True {
        n87 = local write "indexador"(0 ("indexador")) -> ()
        n88 = local write "Manipulando"(FALSE ("Manipulando")) -> ()
      }
    }
    n89 = shared-variable "MARIO\\Variaveis_comuns.lvlib\\Local_da_peca"() -> (w105:i8)  [unwired: 1 in, 1 out]
    n90 = shared-variable "MARIO\\Variaveis_comuns.lvlib\\caminho"(w114) -> ()  [unwired: 1 in, 1 out]
    n91 = call <vilib>:"Set Duty Cycle.vi"("Duty Cycle"=w199, "PWM Ref In"=w201) -> ("PWM Ref Out"=w200:T13)  [unwired: 7 in, 1 out]
    n92 = call <vilib>:"Set Duty Cycle.vi"("Duty Cycle"=w197, "PWM Ref In"=w198) -> ("PWM Ref Out"=w194:T13)  [unwired: 7 in, 1 out]
    n93 = Build Array(w173, w172, w171, w152, w170, "angulo_garra") -> (w169:dbl[])
    "appended array 2" <- w169
    n94 = call "converter_Craig_to_Jonas.vi"("array"=w169) -> ("appended array"=w162:dbl[])
    n95 = Not Equal?(x=w162, y=w149) -> (x != y?=w221:bool[])
    n96 = Or Array Elements(Boolean array=w221) -> (logical OR=w134:bool)
    n97 = case shown="True" w135 {
      tunnel: [w248 FALSE] -> w123
      tunnel: w134 -> [w248 _]
      tunnel: [w247 TRUE ("Actuator")] -> w133
      frame False {
        n98 = local read "Actuator"() -> (w247:bool)
      }
      frame True {
        n99 = Wait (ms)(milliseconds to wait=u32 500) -> ()  [unwired: 1 out]
      }
    }
    n100 = local write "Actuator"(w133) -> ()
    n101 = case shown="True" w125 {
      tunnel: [w243 FALSE ("Actuator")] -> w124
      tunnel: w123 -> [w242 _]
      tunnel: [w242 FALSE] -> w122
      frame False {
        n102 = local read "Actuator"() -> (w243:bool)
      }
      frame True {
        n103 = Wait (ms)(milliseconds to wait=u32 500) -> ()  [unwired: 1 out]
      }
    }
    n104 = local write "Actuator"(w124) -> ()
    n105 = case shown="True" w122 {
      tunnel: [w312 w320] -> w225
      tunnel: w223 -> [w312 w319]
      tunnel: w222 -> [_ w318]
      tunnel: w149 -> [w313 w317]
      tunnel: [w313 w315] -> w157
      tunnel: u32 7 ("ms to wait (braço)") -> [_ w316]
      tunnel: w162 -> [_ w314]
      frame False {
      }
      frame True {
        n106 = for {
          tunnel: w318 -> [w326] mode=indexing
          tunnel: w317 -> [w325] mode=indexing
          tunnel: w316 -> [w323]
          tunnel: [w322] -> w315 mode=indexing
          tunnel: w314 -> [w321] mode=indexing
          shift-right: [w328] -> w320
          shift-left: w319 -> [w327]
          n107 = call "SubVI_Controle_velocidade_servo.vi"("Posição Desejada"=w321, "Posição"=w325, "milliseconds to wait"=w323) -> ("Duty Cycle"=w324:dbl, "Posição"=w322:dbl)  [unwired: 7 in]
          n108 = call <vilib>:"Set Duty Cycle.vi"("error in (no error)"=w327, "Duty Cycle"=w324, "PWM Ref In"=w326) -> ("error out"=w328:errorcluster)  [unwired: 6 in, 1 out]
        }
      }
    }
    n109 = Subtract(x=w162, y=w157) -> (x-y=w220:dbl[])
    n110 = Absolute Value(x=w220) -> (abs(x)=w219:dbl[])
    n111 = local read "ANG_POSI_E_ORIEN_HOME"() -> (w168:dbl[])
    n112 = Array Max & Min(array=w219) -> (max value=w161:dbl)  [unwired: 3 out]
    n113 = local read "Manipulando"() -> (w213:bool)
    n114 = Index Array(array=w157) -> (element #1=w186:dbl, element #2=w185:dbl, element #3=w184:dbl, element #4=w183:dbl, element #5=w182:dbl, element #6=w181:dbl)  [unwired: 6 in]
    n115 = Less?(x=w161, y=1.0) -> (x < y?=w158:bool)
    "Posicao_desejada" <- w158
    n116 = And(x=w158, y=w213) -> (x .and. y?=w212:bool)
    "x .and. y?" <- w212
    n117 = Subtract(x=w168, y=w157) -> (x-y=w210:dbl[])
    n118 = call "converter_Jonas_to_Craig.vi"("theta6Jonas"=w181, "theta1Jonas"=w186, "theta5Jonas"=w182, "theta4Jonas"=w183, "theta3Jonas"=w184, "theta2Jonas"=w185) -> ("theta5Craig"=w176:dbl, "theta4Craig"=w177:dbl, "theta3Craig"=w178:dbl, "theta2Craig"=w179:dbl, "theta6Craig"=w175:dbl, "theta1Craig"=w180:dbl)
    n119 = Absolute Value(x=w210) -> (abs(x)=w209:dbl[])
    n120 = Delete From Array(array=w144, index (row)=w104) -> (deleted portion=w148:dbl[])  [unwired: 2 in, 1 out]
    "subarray" <- w148
    n121 = case shown="False" w212 {
      tunnel: w214 -> [_ w300]
      tunnel: [u32 0 ("ms to wait (braço)") w299] -> w215
      frame False {
      }
      frame True {
        n122 = Increment(x=w300) -> (x+1=w299:u32)
        n123 = Equal?(x=w299, y=u32 1) -> (x = y?=w297:bool)
        n124 = case shown="True" w297 {
          frame False {
          }
          frame True {
            n125 = local read "indexador"() -> (w302:i32)
            n126 = Increment(x=w302) -> (x+1=w301:i32)
            n127 = local write "indexador"(w301) -> ()
          }
        }
      }
    }
    "iterador" <- w215
    n128 = Array Max & Min(array=w209) -> (max value=w208:dbl)  [unwired: 3 out]
    n129 = Build Array(w180, w179, w178, w177, w176, w175) -> (→"CURRENT POSITIONS OF THE MOTORS":dbl[])
    n130 = Matrix Size(0:w144) -> (1:w147:i32)  [unwired: 1 out]
    "number of rows" <- w147
    n131 = Less?(x=w208, y=1.1) -> (x < y?=w192:bool)
    "Está em Home" <- w192
    n132 = Increment(x=w104) -> (x+1=w142:i32)
    n133 = shared-variable "MARIO\\Variaveis_comuns.lvlib\\Braço_pronto"(w192) -> ()  [unwired: 1 in, 1 out]
    n134 = Equal?(x=w142, y=w147) -> (x = y?=w205:bool)
    n135 = case shown="True" w205 {
      tunnel: [w294 FALSE ("Manipulando")] -> w143
      tunnel: w141 -> [w294 _]
      frame False {
      }
      frame True {
      }
    }
    n136 = case shown="True" w141 {
      tunnel: w148 -> [_ w252]
      frame False {
      }
      frame True {
        n137 = local write "POSITION VECTOR"(w252) -> ()
      }
    }
    "Objeto detectado" <- "OK Button"
    "Actuator 2" <- "Actuator"
    "matrix" <- w144
  }
  n138 = Insert Into Array(array=w45, new element #1=w44, new element #2=w36) -> (w43:T13[])  [unwired: 1 in]
  n139 = call "stopContinuous.vi"("error in"=w5, "Slave Address(7 bit)"=w9, "I2C Ref In"=w10) -> ("error out"=w7:errorcluster, "I2C Ref Out"=w8:T5)  [unwired: 7 in]
  n140 = for {
    tunnel: w54 -> [w330]
    tunnel: w43 -> [w329] mode=indexing
    n141 = call <vilib>:"Close.vi"("error in (no error)"=w330, "PWM Ref In"=w329) -> ()  [unwired: 9 in, 1 out]
  }
  n142 = call <vilib>:"Close.vi"("error in (no error)"=w7, "I2C Ref In"=w8) -> ("error out"=→"error out":errorcluster)  [unwired: 9 in]
  "indexador" <- 0
